vi "Project Initializer - Rename Folder.vi"(7 "Project Path":path, 8 "error in (no error)":errorcluster, 9 "Target Project Name":string, 10 "Source Project Name":string, 11 "Folder Suffix":string) -> (0 "error out":errorcluster, 3 "New Folder Path":path)   [LabVIEW 2022 SP3]
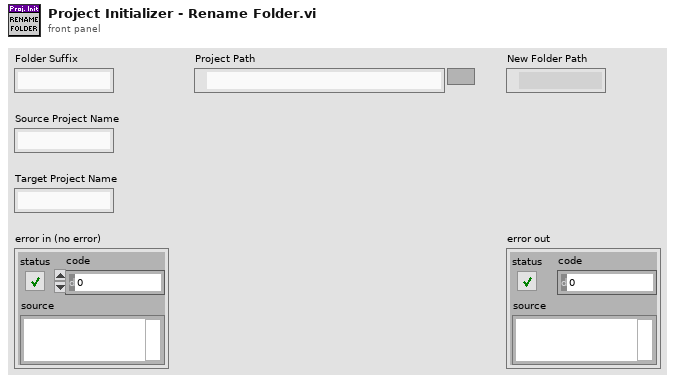
[diagram p1: front panel]
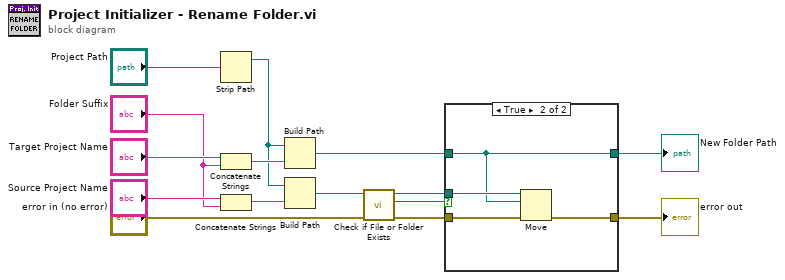
[diagram p0: block diagram]
diagram:
  n1 = Strip Path(path="Project Path") -> (stripped path=w2:path)  [unwired: 1 out]
  n2 = Concatenate Strings("Target Project Name", "Folder Suffix") -> (w11:string)
  n3 = Concatenate Strings("Source Project Name", "Folder Suffix") -> (w10:string)
  n4 = Build Path(base path=w2, name or relative path=w11) -> (appended path=w13:path)
  n5 = Build Path(base path=w2, name or relative path=w10) -> (appended path=w6:path)
  n6 = call <vilib>:"Check if File or Folder Exists.vi"("error in (no error)"="error in (no error)", "path"=w6) -> ("error out"=w7:errorcluster, "file or folder exists?"=w4:bool, "dup path"=w5:path)  [unwired: 7 in]
  n7 = case shown="True" w4 {
    tunnel: w13 -> [w16 w18]
    tunnel: w5 -> [_ w21]
    tunnel: [w17 w20] -> w9
    tunnel: w7 -> [w17 w19]
    tunnel: [w16 w18] -> w1
    frame False {
    }
    frame True {
      n8 = Move(source path=w21, error in=w19, 10:w18) -> (error out=w20:errorcluster)  [unwired: 2 in, 2 out]
    }
  }
  "error out" <- w9
  "New Folder Path" <- w1
